vi "Stop Motor Torque.vi"(6 "error in":errorcluster, 8 "MaxRead":i32, 9 "Channel in":u16) -> (0 "error out":errorcluster, 1 "Messages":T2(array[cluster]) {"DATA[0]" format="%.0x"; "DATA[2]" format="%.0x"; "DATA[3]" format="%.0x"; "DATA[4]" format="%.0x"}, 2 "Pass":bool, 3 "Channel out":u16)   [LabVIEW 2023]
uses:
  df35a301-8fcb-495c-91e3-c82146f18b8b.vi
  9e829622-24b2-4c22-b142-2813b4f57ddd.vi
  0e3a88ba-a1c3-4589-a0b0-66c397795f2f.vi
  2ad30504-fef7-4a6b-a16d-0a474ce5601d.vi
  e99ada8f-d09f-4018-ada1-fc308b247a31.vi
  Communication/PCAN2023/PCAN API.lvlib
panel:
  out "logical AND 2":bool
  out "Passed":bool
  out "logical AND":bool
  out "x = y?":bool
  out "Last Message 3":T1
  out "Last Message 2":T1
  out "Last Message":T1 {"DATA[0]" format="%.0x"}
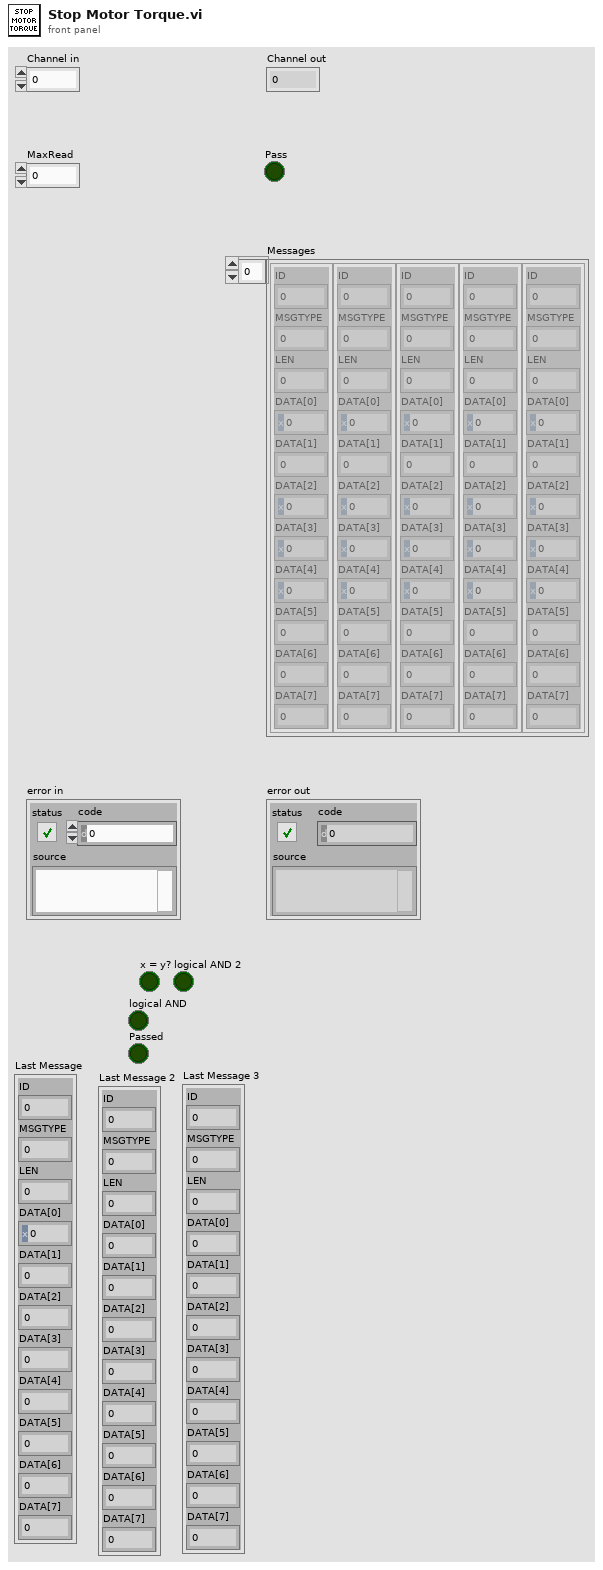
[diagram p1: front panel]
types:
  T1 = cluster{"ID":u32, "MSGTYPE":u8, "LEN":u8, "DATA[0]":u8, "DATA[1]":u8, "DATA[2]":u8, "DATA[3]":u8, "DATA[4]":u8, "DATA[5]":u8, "DATA[6]":u8, "DATA[7]":u8}
  T2 = cluster{"ID":u32, "MSGTYPE":u8, "LEN":u8, "DATA[0]":u8, "DATA[1]":u8, "DATA[2]":u8, "DATA[3]":u8, "DATA[4]":u8, "DATA[5]":u8, "DATA[6]":u8, "DATA[7]":u8}[]
  T3 = cluster{"ID":bool, "MSGTYPE":bool, "LEN":bool, "DATA[0]":bool, "DATA[1]":bool, "DATA[2]":bool, "DATA[3]":bool, "DATA[4]":bool, "DATA[5]":bool, "DATA[6]":bool, "DATA[7]":bool}
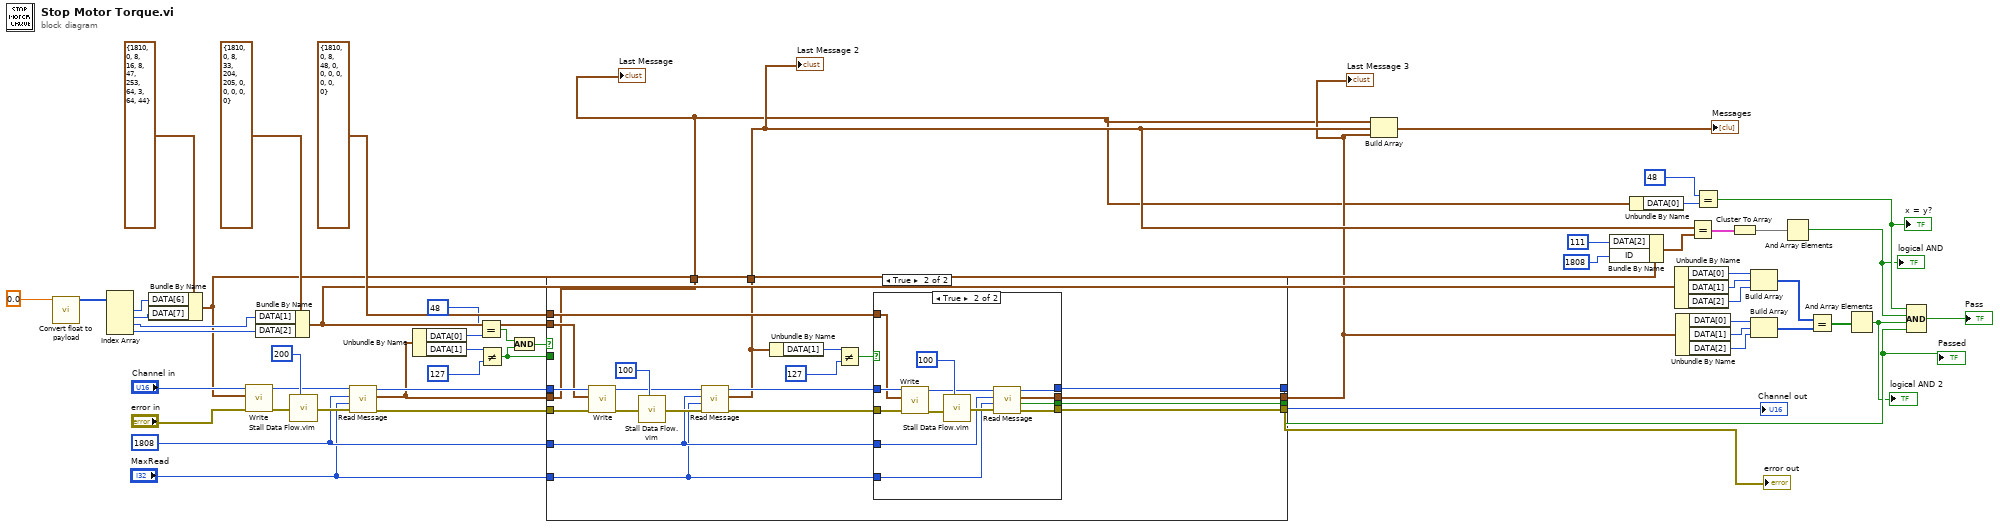
[diagram p0: block diagram]
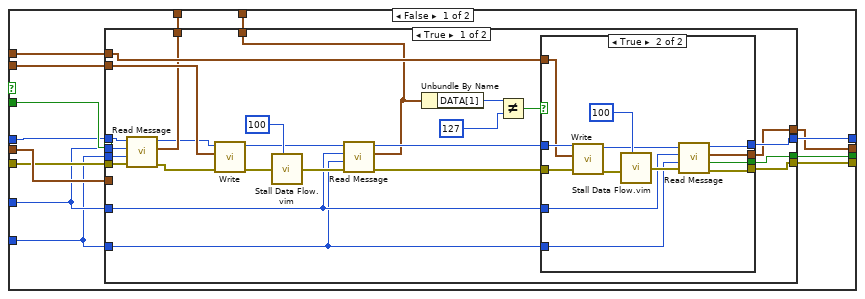
[diagram p2: hidden frame]
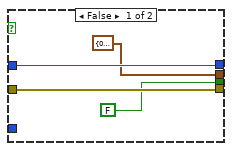
[diagram p3: hidden frame]
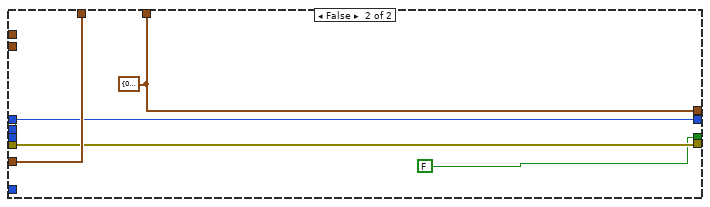
[diagram p4: hidden frame]
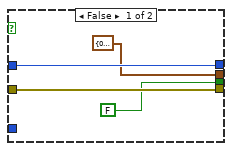
[diagram p5: hidden frame]
diagram:
  w19 = u32 1808 ("ID")
  n1 = call "Convert float to payload.vi"("FloatNumber"=sgl 0.0) -> ("Converted Payload"=w50:u8[])  [unwired: 18 in]
  n2 = Index Array(array=w50) -> (element #1=w49:u8, element #2=w48:u8, element #3=w46:u8, element #4=w45:u8)  [unwired: 4 in]
  n3 = Bundle By Name(cluster=T1 {"ID"=1810, "MSGTYPE"=0, "LEN"=8, "DATA[0]"=16, "DATA[1]"=8, "DATA[2]"=47, "DATA[3]"=253, "DATA[4]"=64, "DATA[5]"=3, "DATA[6]"=64, "DATA[7]"=44} ("MessageBuffer"), "DATA[6]"=w49, "DATA[7]"=w48) -> (w41:T1)
  n4 = call "Write.vi"("error in"="error in", "MessageBuffer"=w41, "Channel"="Channel in") -> ("error out"=w55:errorcluster, "Channel out"=w23:u16)  [unwired: 5 in, 2 out]
  n5 = Bundle By Name(cluster=T1 {"ID"=1810, "MSGTYPE"=0, "LEN"=8, "DATA[0]"=33, "DATA[1]"=204, "DATA[2]"=205, "DATA[3]"=0, "DATA[4]"=0, "DATA[5]"=0, "DATA[6]"=0, "DATA[7]"=0} ("MessageBuffer"), "DATA[1]"=w46, "DATA[2]"=w45) -> (w39:T1)
  n6 = call "Stall Data Flow.vim"("value in"=w55, "milliseconds to wait"=u32 200) -> ("value out"=w21:errorcluster)  [unwired: 1 out]
  n7 = call "Read Message.vi"("error in"=w21, "MaxRead"="MaxRead", "ID"=w19, "Channel in"=w23) -> ("error out"=w20:errorcluster, "Last Message"=w2:T1, "Channel out"=w22:u16)  [unwired: 3 in, 2 out]
  n8 = Unbundle By Name(w2) -> ("DATA[0]"=w7:u8, "DATA[1]"=w24:u8)
  n9 = Equal?(x=u8 48, y=w7) -> (x = y?=w5:bool)
  n10 = Not Equal?(x=w24, y=u8 127) -> (x != y?=w3:bool)
  n11 = And(x=w5, y=w3) -> (x .and. y?=w4:bool)
  n12 = case shown="True" w4 {
    tunnel: w22 -> [w65 w137]
    tunnel: w20 -> [w62 w136]
    tunnel: T1 {"ID"=1810, "MSGTYPE"=0, "LEN"=8, "DATA[0]"=48, "DATA[1]"=0, "DATA[2]"=0, "DATA[3]"=0, "DATA[4]"=0, "DATA[5]"=0, "DATA[6]"=0, "DATA[7]"=0} ("MessageBuffer") -> [w66 w134]
    tunnel: w39 -> [w67 w133]
    tunnel: [w69 w132] -> w9
    tunnel: [w58 w131] -> w31
    tunnel: [w59 w130] -> w30
    tunnel: [w57 w129] -> w12
    tunnel: [w70 w121] -> w13
    tunnel: w19 -> [w61 w120]
    tunnel: "MaxRead" -> [w60 w119]
    tunnel: w3 -> [w68 _]
    tunnel: w2 -> [w63 w118]
    tunnel: [w64 w118] -> w1
    frame False {
      n13 = case shown="True" w68 {
        tunnel: [w84 w116] -> w70
        tunnel: [w71 FALSE] -> w69
        tunnel: w67 -> [w86 _]
        tunnel: w66 -> [w85 _]
        tunnel: w65 -> [w83 w115]
        tunnel: [w82 w117] -> w64
        tunnel: w63 -> [_ w117]
        tunnel: w62 -> [w81 w114]
        tunnel: w61 -> [w80 _]
        tunnel: w60 -> [w79 _]
        tunnel: w61 -> [w76 _]
        tunnel: w60 -> [w75 _]
        tunnel: [w74 w115] -> w59
        tunnel: [w73 w114] -> w58
        tunnel: [w72 w116] -> w57
        frame True {
          n14 = call "Read Message.vi"("error in"=w81, "MaxRead"=w79, "ID"=w80, "Channel in"=w83) -> ("error out"=w78:errorcluster, "Last Message"=w82:T1, "Channel out"=w77:u16)  [unwired: 3 in, 2 out]
          n15 = call "Write.vi"("error in"=w78, "MessageBuffer"=w86, "Channel"=w77) -> ("error out"=w95:errorcluster, "Channel out"=w90:u16)  [unwired: 5 in, 2 out]
          n16 = call "Stall Data Flow.vim"("value in"=w95, "milliseconds to wait"=u32 100) -> ("value out"=w87:errorcluster)  [unwired: 1 out]
          n17 = call "Read Message.vi"("error in"=w87, "MaxRead"=w75, "ID"=w76, "Channel in"=w90) -> ("error out"=w88:errorcluster, "Last Message"=w84:T1, "Channel out"=w89:u16)  [unwired: 3 in, 2 out]
          n18 = Unbundle By Name(w84) -> ("DATA[1]"=w92:u8)
          n19 = Not Equal?(x=w92, y=u8 127) -> (x != y?=w91:bool)
          n20 = case shown="True" w91 {
            tunnel: w89 -> [w99 w112]
            tunnel: w88 -> [w98 w111]
            tunnel: w85 -> [_ w110]
            tunnel: [FALSE w103] -> w71
            tunnel: [w98 w104] -> w73
            tunnel: [w99 w106] -> w74
            tunnel: [T1 {"ID"=0, "MSGTYPE"=0, "LEN"=0, "DATA[0]"=0, "DATA[1]"=0, "DATA[2]"=0, "DATA[3]"=0, "DATA[4]"=0, "DATA[5]"=0, "DATA[6]"=0, "DATA[7]"=0} ("MessageBuffer out") w102] -> w72
            tunnel: w76 -> [_ w101]
            tunnel: w75 -> [_ w100]
            frame False {
            }
            frame True {
              n21 = call "Write.vi"("error in"=w111, "MessageBuffer"=w110, "Channel"=w112) -> ("error out"=w109:errorcluster, "Channel out"=w107:u16)  [unwired: 5 in, 2 out]
              n22 = call "Stall Data Flow.vim"("value in"=w109, "milliseconds to wait"=u32 100) -> ("value out"=w105:errorcluster)  [unwired: 1 out]
              n23 = call "Read Message.vi"("error in"=w105, "MaxRead"=w100, "ID"=w101, "Channel in"=w107) -> ("error out"=w104:errorcluster, "Passed"=w103:bool, "Last Message"=w102:T1, "Channel out"=w106:u16)  [unwired: 3 in, 1 out]
            }
          }
        }
        frame False {
          w116 = T1 {"ID"=0, "MSGTYPE"=0, "LEN"=0, "DATA[0]"=0, "DATA[1]"=0, "DATA[2]"=0, "DATA[3]"=0, "DATA[4]"=0, "DATA[5]"=0, "DATA[6]"=0, "DATA[7]"=0} ("MessageBuffer out")
        }
      }
    }
    frame True {
      n24 = call "Write.vi"("error in"=w136, "MessageBuffer"=w133, "Channel"=w137) -> ("error out"=w138:errorcluster, "Channel out"=w125:u16)  [unwired: 5 in, 2 out]
      n25 = call "Stall Data Flow.vim"("value in"=w138, "milliseconds to wait"=u32 100) -> ("value out"=w122:errorcluster)  [unwired: 1 out]
      n26 = call "Read Message.vi"("error in"=w122, "MaxRead"=w119, "ID"=w120, "Channel in"=w125) -> ("error out"=w123:errorcluster, "Last Message"=w121:T1, "Channel out"=w124:u16)  [unwired: 3 in, 2 out]
      n27 = Unbundle By Name(w121) -> ("DATA[1]"=w127:u8)
      n28 = Not Equal?(x=w127, y=u8 127) -> (x != y?=w126:bool)
      n29 = case shown="True" w126 {
        tunnel: w124 -> [w142 w155]
        tunnel: w123 -> [w141 w154]
        tunnel: w134 -> [_ w153]
        tunnel: [FALSE w146] -> w132
        tunnel: [w141 w147] -> w131
        tunnel: [w142 w149] -> w130
        tunnel: [T1 {"ID"=0, "MSGTYPE"=0, "LEN"=0, "DATA[0]"=0, "DATA[1]"=0, "DATA[2]"=0, "DATA[3]"=0, "DATA[4]"=0, "DATA[5]"=0, "DATA[6]"=0, "DATA[7]"=0} ("MessageBuffer out") w145] -> w129
        tunnel: w120 -> [_ w144]
        tunnel: w119 -> [_ w143]
        frame False {
        }
        frame True {
          n30 = call "Write.vi"("error in"=w154, "MessageBuffer"=w153, "Channel"=w155) -> ("error out"=w152:errorcluster, "Channel out"=w150:u16)  [unwired: 5 in, 2 out]
          n31 = call "Stall Data Flow.vim"("value in"=w152, "milliseconds to wait"=u32 100) -> ("value out"=w148:errorcluster)  [unwired: 1 out]
          n32 = call "Read Message.vi"("error in"=w148, "MaxRead"=w143, "ID"=w144, "Channel in"=w150) -> ("error out"=w147:errorcluster, "Passed"=w146:bool, "Last Message"=w145:T1, "Channel out"=w149:u16)  [unwired: 3 in, 1 out]
        }
      }
    }
  }
  "error out" <- w31
  "Channel out" <- w30
  "Last Message" <- w1
  "Last Message 2" <- w13
  "Last Message 3" <- w12
  "Passed" <- w9
  n33 = Build Array(w1, w13, w12) -> (→"Messages":T2)
  n34 = Bundle By Name(cluster=w41, "DATA[2]"=u8 111 ("x"), "ID"=u32 1808 ("x")) -> (w16:T1)
  n35 = Unbundle By Name(w1) -> ("DATA[0]"=w43:u8)
  n36 = Unbundle By Name(w39) -> ("DATA[0]"=w35:u8, "DATA[1]"=w34:u8, "DATA[2]"=w33:u8)
  n37 = Unbundle By Name(w12) -> ("DATA[0]"=w38:u8, "DATA[1]"=w37:u8, "DATA[2]"=w36:u8)
  n38 = Equal?(x=w13, y=w16) -> (x = y?=w29:T3)
  n39 = Equal?(x=u8 48, y=w43) -> (x = y?=w11:bool)
  "x = y?" <- w11
  n40 = Cluster To Array(cluster=w29) -> (array=w28:bool[])
  n41 = Build Array(w35, w34, w33) -> (w15:u8[])
  n42 = Build Array(w38, w37, w36) -> (w14:u8[])
  n43 = And Array Elements(Boolean array=w28) -> (logical AND=w10:bool)
  "logical AND" <- w10
  n44 = Equal?(x=w15, y=w14) -> (x = y?=w32:bool[])
  n45 = And Array Elements(Boolean array=w32) -> (logical AND=w8:bool)
  "logical AND 2" <- w8
  n46 = Compound Arithmetic op=AND(w11, w10, w8, w9) -> (→"Pass":bool)
